vi "DELETE DAQ.TimedLoop.vi"(8 "error in (no error)":errorcluster, 11 "DAQmx in":refnum<class "DAQmx.lvclass">) -> (0 "error out":errorcluster, 3 "DAQmx out":refnum<class "DAQmx.lvclass">)   [LabVIEW 2019]
uses:
  DAQmx/DAQmx.lvclass
  <vilib>/Platform/TimedLoop/XDataNode/wakeup.ctl
  <vilib>/Platform/TimedLoop/XDataNode/XDNodeRunTimeDep.lvlib
  <vilib>/Platform/TimedLoop/XDataNode/nitl_modes.ctl
  <vilib>/Platform/TimedLoop/XDataNode/timing_clust.ctl
  <vilib>/platform/TimedLoop/XDataNode/XDataNode.xnode
  Instrument.DAQ/Instrument.DAQ.lvclass
  Generator/Generator.lvclass
  Instrument.DAQ/Typedefs/Set State-enum.ctl
  <vilib>/JKI/JKI SMO/SMO/SMO.lvclass
  C:/Program Files (x86)/National Instruments/LabVIEW 2019/vi.lib/JKI/JKI SMO/SMO/SMO.lvclass
panel:
  out "Lockin":u32
  out "AO/AI":u32
  out "generate":u32
  # "!!!!!!!!!!!!!!!!!!!!!!!!!!!!!!!!!!!!!!!!!!!!!!!!!!!!!!!!!!!!!!!!!!!!!!!!\nTHIS IS AN EXPERIMENTAL BLOCKING CALL TO:\nGenerate\nRead/Write\nDSP\nIt should listen to events that change AO or REF Channels.\nInside there is a timed loop that will not stop unless it receives events for Set State = stop; SMO Stop; or SMO error\n!!!!!!!!!!!!!!!!!!!!!!!!!!!!!!!!!!!!!!!!!!!!!!!!!!!!!!!!!!!!!!!!!!!!!"
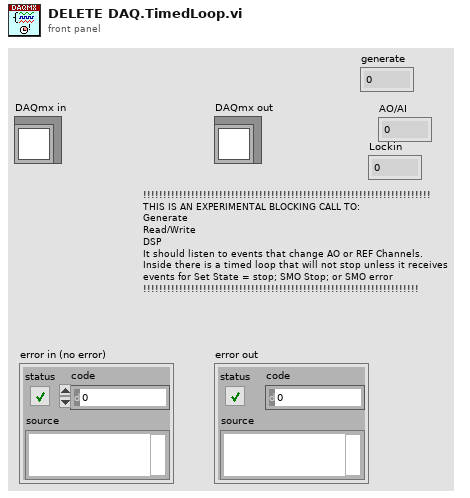
[diagram p1: front panel]
types:
  T1 = typedef "Instrument.Lockin.lvlib/Instrument.DAQ.lvclass/Set State-enum.ctl" = enum16{"start", "stop", "reset", "start sweep", "stop sweep"}
  T2 = typedef "XDNodeRunTimeDep.lvlib/timing_clust.ctl" = cluster{"Expected End [f-1]":u64, "Actual End [f-1]":u64, "Finished Late? [f-1]":bool, "Expected End [i-1]":u64, "Actual End [i-1]":u64, "Finished Late? [i-1]":bool, "Expected Start [i]":u64, "Actual Start [i]":u64, "Expected Start [f]":u64, "Actual Start [f]":u64, "Source Name":string, "Structure Name":string, "Period":i64, "Deadline":i64, "Offset":i64, "Start":i64, "Priority":i32, "Timeout":i32, "Mode":T3, "Wakeup Reason":T4, "Error":errorcluster, "Source Type":string, "Secondary Source Type":string, "Global End Time":u64, "Global Start Time":u64, "Frame Duration":u64, "Iteration Duration":u64, "Assigned CPU":i32, "I/O Scan Engine Mode":u32}
  T3 = typedef "XDNodeRunTimeDep.lvlib/nitl_modes.ctl" = enum32{"No Change", "Process missed periods, maintain original phase", "Discard missed periods, maintain original phase", "Process missed periods, ignore original phase", "Discard missed periods, ignore original phase"}
  T4 = typedef "XDNodeRunTimeDep.lvlib/wakeup.ctl" = enum32{"Normal", "Aborted", "Asynchronous wakeup", "Timing source error", "Timed loop error", "Timeout"}
  T5 = typedef "SMO.lvclass/Protected Events.ctl" = cluster{"StopProcesses":refnum<user-event>, "AbortProcesses":refnum<user-event>, "Config Changed":refnum<user-event>, "Dependency":refnum<user-event>}
  T6 = typedef "Instrument.Lockin.lvlib/Instrument.DAQ.lvclass/PrivateEvents--Cluster.ctl" = cluster{"setAOconfig":refnum<user-event>, "setAIconfig":refnum<user-event>, "setAO":refnum<user-event>, "setREF":refnum<user-event>, "setSampling":refnum<user-event>, "setState":refnum<user-event>, "setInputGain":refnum<user-event>, "setOutputGain":refnum<user-event>, "setSweep":refnum<user-event>, "measureOffset":refnum<user-event>, "zeroOffset":refnum<user-event>, "setPreFilter":refnum<user-event>, "autoConfigureDAQ":refnum<user-event>, "setCalibration":refnum<user-event>, "setAI":refnum<user-event>, "zeroPhase":refnum<user-event>, "setAmplitudeLimit":refnum<user-event>, "setLinkFrequencies":refnum<user-event>, "showUI":refnum<user-event>, "setInputOffset":refnum<user-event>, "setDCLimit":refnum<user-event>}
  T7 = typedef "Instrument.Lockin.lvlib/Instrument.DAQ.lvclass/Results--Cluster.ctl" = cluster{"Time Stamp":timestamp, "Results (Dictionary)":cluster{"key":string, "value":dbl}[]}
  T8 = typedef "Instrument.Lockin.lvlib/Instrument.DAQ.lvclass/AO.Channel--Cluster--Array.ctl" = T9[]
  T9 = typedef "Instrument.Lockin.lvlib/Instrument.DAQ.lvclass/AO.Channel--Cluster.ctl" = cluster{"Enable?":bool, "Channel":i32, "Amplitude":dbl, "Offset":dbl, "Frequency":dbl, "Phase":dbl, "Function":T10, "Sweeping?":bool, "Limit AC":bool, "Limit DC?":bool}
  T10 = typedef "Instrument.Lockin.lvlib/Instrument.DAQ.lvclass/AO.Channel.Function--Enum.ctl" = enum16{"Sine", "Triangle", "Square"}
  T11 = typedef "Instrument.Lockin.lvlib/Instrument.DAQ.lvclass/REF.Channel--Cluster--Array.ctl" = T12[]
  T12 = typedef "Instrument.Lockin.lvlib/Instrument.DAQ.lvclass/REF.Channel--Cluster.ctl" = cluster{"Enable?":bool, "Channel":i32, "Frequency":dbl, "Phase":dbl, "TC":dbl, "Roll-Off":i32}
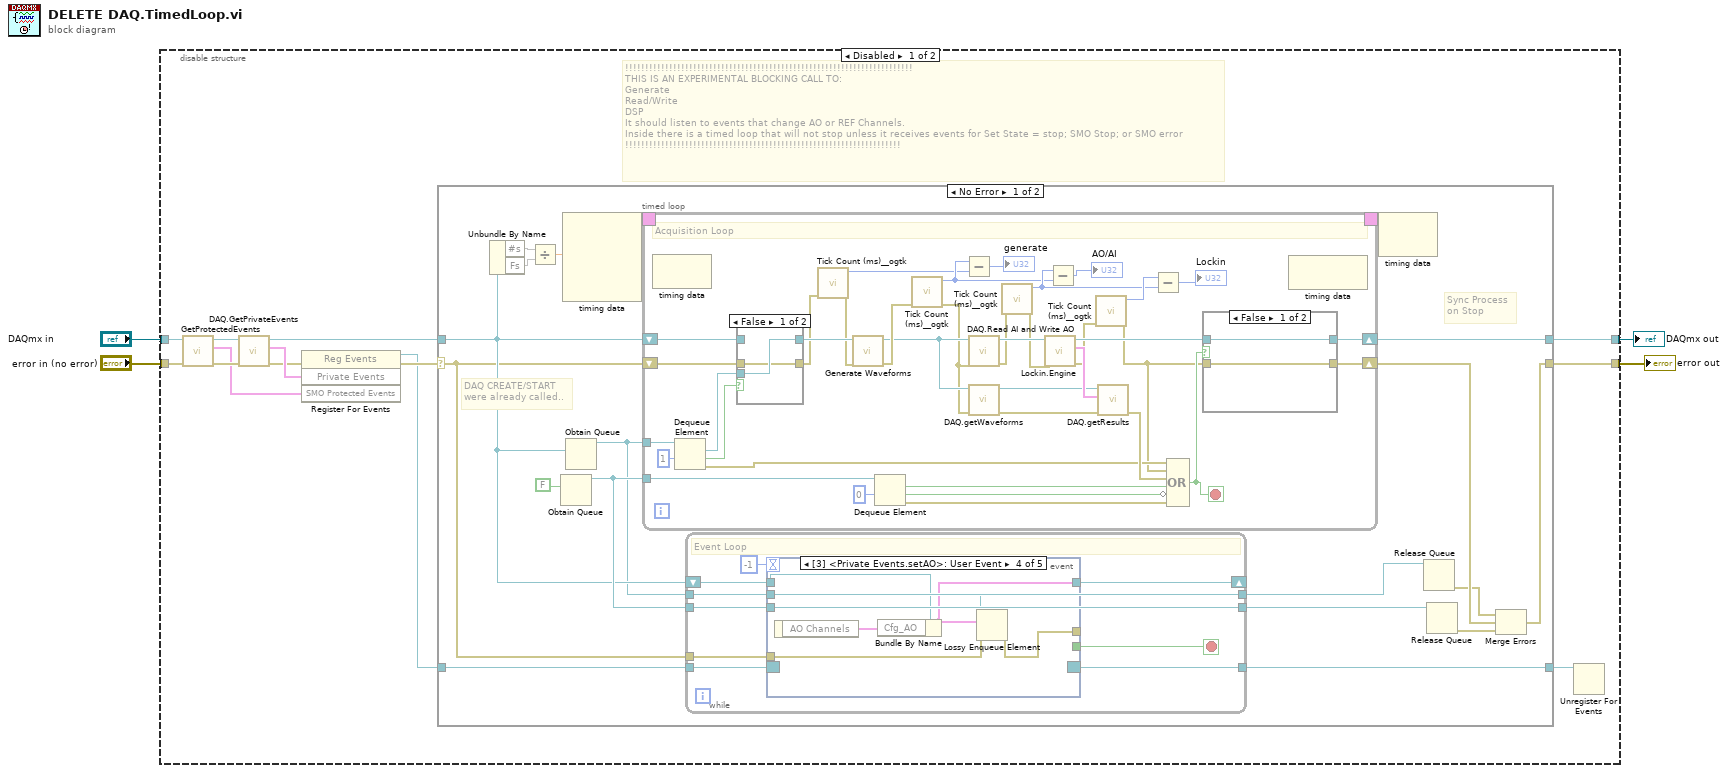
[diagram p0: block diagram]
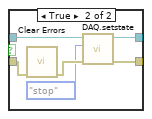
[diagram p2: hidden frame]
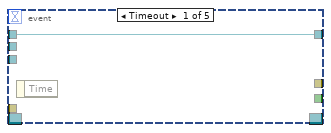
[diagram p4: hidden frame]
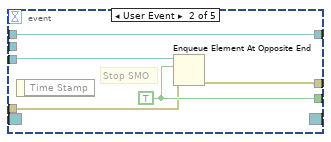
[diagram p5: hidden frame]
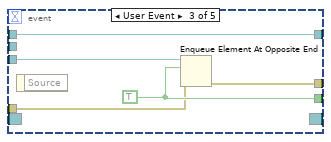
[diagram p6: hidden frame]
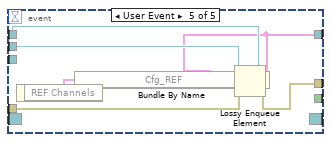
[diagram p7: hidden frame]
diagram:
  n1 = disable-structure shown="Disabled" {
    disable-tunnel: "DAQmx in" -> [w15 w129]
    disable-tunnel: [w14 w129] -> w3
    disable-tunnel: "error in (no error)" -> [w13 w128]
    disable-tunnel: [w5 w128] -> w1
    frame Disabled {
      # "!!!!!!!!!!!!!!!!!!!!!!!!!!!!!!!!!!!!!!!!!!!!!!!!!!!!!!!!!!!!!!!!!!!!!!!!\nTHIS IS AN EXPERIMENTAL BLOCKING CALL TO:\nGenerate\nRead/Write\nDSP\nIt should listen to events that change AO or REF Channels.\nInside there is a timed loop that will not stop unless it receives events for Set State = stop; SMO Stop; or SMO error\n!!!!!!!!!!!!!!!!!!!!!!!!!!!!!!!!!!!!!!!!!!!!!!!!!!!!!!!!!!!!!!!!!!!!!"
      n2 = call <vilib>:"GetProtectedEvents.vi"("error in (no error)"=w13, "SMO"=w15) -> ("error out"=w11:errorcluster, "SMO Protected Events"=w10:T5, "SMO out"=w12:refnum<class "SMO.lvclass">)  [unwired: 7 in]
      n3 = call "DAQ.GetPrivateEvents.vi"("error in (no error)"=w11, "Instrument.DAQ"=w12) -> ("error out"=w7:errorcluster, "Private Events"=w9:T6, "Instrument.DAQ out"=w8:refnum<class "Instrument.DAQ.lvclass">)  [unwired: 7 in]
      n4 = register-events(error in=w7, w9, w10) -> (reference out=w6:refnum<event-registration>, error out=w17:errorcluster)  [unwired: 1 in]
      n5 = case shown="No Error" w17 {
        selector: w17 -> [w22 w125]
        tunnel: w8 -> [w23 w126]
        tunnel: w6 -> [w34 w127]
        tunnel: [w28 w125] -> w5
        tunnel: [w33 w127] -> w16
        tunnel: [w19 w126] -> w14
        frame No Error {
          # "DAQ CREATE/START\nwere already called.."
          # "Sync Process\non Stop"
          n6 = Unbundle By Name(w23) -> ("#s"=w27, "Fs"=w25)
          n7 = Divide(x=w27, y=w25) -> (x/y=w26:dbl)
          n8 = Obtain Queue(element data type=FALSE) -> (queue out=w31:refnum<queue>)  [unwired: 4 in, 2 out]
          n9 = node-c288(w26) -> (w36:T2)  [unwired: 3 in]
          n10 = Obtain Queue(element data type=w23) -> (queue out=w18:refnum<queue>)  [unwired: 4 in, 2 out]
          n11 = timed-loop {
            timing: w36 -> [_]
            timing-out: [_] -> w35
            tunnel: w31 -> [w74]
            shift-right: [w56] -> w19
            shift-left: w23 -> [w61]
            shift-right: [w55] -> w24
            shift-left: w22 -> [w60]
            tunnel: w18 -> [w66]
            stop <- w58 stop-if-true
            # "Acquisition Loop"
            n12 = node-c288() -> ()  [unwired: 1 in, 1 out]
            n13 = Dequeue Element(queue=w66, timeout in ms (-1)=1) -> (element=w63:refnum<class "Instrument.DAQ.lvclass">, timed out?=w64:bool, error out=w59:errorcluster)  [unwired: 1 in, 1 out]
            n14 = case shown="False" w64 {
              tunnel: w63 -> [w84 _]
              tunnel: [w84 w86] -> w62
              tunnel: w61 -> [_ w86]
              tunnel: w60 -> [w83 w85]
              tunnel: [w83 w85] -> w54
              frame False {
              }
              frame True {
              }
            }
            n15 = call <userlib>:"Tick Count (ms)__ogtk.vi"("error in (no error)"=w54) -> ("error out"=w53:errorcluster, "millisecond timer value"=w44:u32)  [unwired: 9 in]
            n16 = call "Generate Waveforms.vi"("error in (no error)"=w53, "Generator.lvclass"=w62) -> ("error out"=w52:errorcluster, "Generator.lvclass"=w40:refnum<class "Generator.lvclass">)  [unwired: 5 in, 3 out]
            n17 = Dequeue Element(queue=w74, timeout in ms (-1)=0) -> (element=w72:bool, timed out?=w71:bool, error out=w70:errorcluster)  [unwired: 1 in, 1 out]
            n18 = call <userlib>:"Tick Count (ms)__ogtk.vi"("error in (no error)"=w52) -> ("error out"=w39:errorcluster, "millisecond timer value"=w45:u32)  [unwired: 9 in]
            n19 = Subtract(x=w45, y=w44) -> (x-y=→"generate":u32)
            n20 = call "DAQ.Read AI and Write AO.vi"("error in (no error)"=w39, "Instrument.DAQ in"=w40) -> ("error out"=w51:errorcluster, "Instrument.DAQ out"=w69:refnum<class "Instrument.DAQ.lvclass">)  [unwired: 8 in]
            n21 = call "DAQ.getWaveforms.vi"("error in (no error)"=w39, "Instrument.DAQ"=w40) -> ("error out"=w38:errorcluster, "Instrument.DAQ"=w37:refnum<class "Instrument.DAQ.lvclass">)  [unwired: 8 in]
            n22 = call <userlib>:"Tick Count (ms)__ogtk.vi"("error in (no error)"=w51) -> ("error out"=w50:errorcluster, "millisecond timer value"=w46:u32)  [unwired: 9 in]
            n23 = call "Lockin.Engine.vi"("error in (no error)"=w50, "Instrument.DAQ"=w69) -> ("error out"=w49:errorcluster, "<Results> (X,Y,R,Theta,Mean)"=w68:T7, "Instrument.DAQ out"=w57:refnum<class "Instrument.DAQ.lvclass">)  [unwired: 7 in]
            n24 = Subtract(x=w46, y=w45) -> (x-y=→"AO/AI":u32)
            n25 = call <userlib>:"Tick Count (ms)__ogtk.vi"("error in (no error)"=w49) -> ("error out"=w48:errorcluster, "millisecond timer value"=w47:u32)  [unwired: 9 in]
            n26 = call "DAQ.getResults.vi"("error in (no error)"=w38, "Results"=w68, "Instrument.DAQ"=w37) -> ("error out"=w67:errorcluster)  [unwired: 7 in, 1 out]
            n27 = Subtract(x=w47, y=w46) -> (x-y=→"Lockin":u32)
            n28 = Compound Arithmetic op=OR(w59, w48, w67, w72, invert w71, w70) -> (w58:bool)
            n29 = case shown="False" w58 {
              tunnel: w57 -> [w75 w82]
              tunnel: [w75 w81] -> w56
              tunnel: [w76 w80] -> w55
              tunnel: w48 -> [w76 w78]
              frame False {
              }
              frame True {
                n30 = call <vilib>:"Clear Errors.vi"("error in (no error)"=w78) -> ("error out"=w79:errorcluster)  [unwired: 5 in, 1 out]
                n31 = call "DAQ.setstate.vi"("error in (no error)"=w79, "setState"=Set_State-enum."stop", "Instrument.DAQ"=w82) -> ("error out"=w80:errorcluster, "Instrument.DAQ out"=w81:refnum<class "Instrument.DAQ.lvclass">)  [unwired: 7 in]
              }
            }
            n32 = node-c288() -> ()  [unwired: 1 in, 1 out]
          }
          n33 = while {
            tunnel: w34 -> [w99]
            tunnel: [w98] -> w33
            shift-right: [w95] -> _
            shift-left: w23 -> [w96]
            tunnel: w22 -> [w94]
            tunnel: w18 -> [w93]
            tunnel: [w93] -> w21
            tunnel: w31 -> [w92]
            tunnel: [w92] -> w30
            stop <- w97 stop-if-true
            # "Event Loop"
            n34 = event shown="[3] <Private Events.setAO>: User Event" {
              selector: w99 -> [_ _ _ _ _]
              dyn-events: [_ _ _ _ _] -> w98
              timeout: -1 -> [_ _ _ _ _]
              tunnel: [_ w105 w108 _ _] -> w97
              tunnel: w92 -> [_ w106 w111 _ _]
              tunnel: [_ w102 w110 w116 w122] -> _
              tunnel: w96 -> [w101 w104 w109 w115 w121]
              tunnel: [w101 w104 w109 w113 w119] -> w95
              tunnel: w94 -> [_ w103 w107 w112 w118]
              tunnel: w93 -> [_ _ _ w117 w123]
              event Timeout {
                n35 = event-data() -> ()  [unwired: 1 in, 1 out]
              }
              event User Event {
                w105 = TRUE
                # "Stop SMO"
                n36 = event-data() -> ()  [unwired: 1 in, 1 out]
                n37 = Enqueue Element At Opposite End(queue=w106, element=w105, error in (no error)=w103) -> (error out=w102:errorcluster)  [unwired: 1 in, 2 out]
              }
              event User Event {
                w108 = TRUE
                n38 = event-data() -> ()  [unwired: 1 in, 1 out]
                n39 = Enqueue Element At Opposite End(queue=w111, element=w108, error in (no error)=w107) -> (error out=w110:errorcluster)  [unwired: 1 in, 2 out]
              }
              event User Event {
                n40 = event-data() -> ("AO Channels"=w114:T8)  [unwired: 1 in]
                n41 = Bundle By Name(cluster=w115, "Cfg_AO"=w114) -> (w113:cluster{})
                n42 = Lossy Enqueue Element(queue=w117, element=w113, error in (no error)=w112) -> (error out=w116:errorcluster)  [unwired: 3 out]
              }
              event User Event {
                n43 = event-data() -> ("REF Channels"=w120:T11)  [unwired: 1 in]
                n44 = Bundle By Name(cluster=w121, "Cfg_REF"=w120) -> (w119:cluster{})
                n45 = Lossy Enqueue Element(queue=w123, element=w119, error in (no error)=w118) -> (error out=w122:errorcluster)  [unwired: 3 out]
              }
            }
          }
          n46 = node-c288(w35) -> ()  [unwired: 1 out]
          n47 = Release Queue(queue=w21) -> (error out=w20:errorcluster)  [unwired: 2 in, 2 out]
          n48 = Release Queue(queue=w30) -> (error out=w29:errorcluster)  [unwired: 2 in, 2 out]
          n49 = Merge Errors(w20, w24, w29) -> (w28:errorcluster)
        }
        frame Error {
        }
      }
      n50 = Unregister For Events(event registration refnum=w16) -> ()  [unwired: 1 in, 1 out]
    }
    frame Enabled {
    }
  }
  "DAQmx out" <- w3
  "error out" <- w1
